vi "ReadEnricoData.vi"(0 "file path":path) -> (1 "Real Graph Enrico":cluster{"Signal":dbl[], "Signal":dbl[]}, 2 "Real Error bars":cluster{dbl[], dbl[]}(graph), 3 "Imaginary Graph Enrico":cluster{"Signal":dbl[], "Signal":dbl[]}, 4 "Imaginary Error bars":cluster{dbl[], dbl[]}(graph))   [LabVIEW 2011]
uses:
  <vilib>/Platform/storage/lvStorage.llb/_openStorageWithRootAutoDetect.vi
  <vilib>/Platform/storage/lvStorage.llb/xStorage/xStorageSupp/ErrorOut.vi
  <vilib>/Platform/storage/lvStorage.llb/_queryPropDateTime.vi
  <vilib>/Platform/storage/lvStorage.llb/_queryGenericObjects.vi
  <vilib>/Platform/storage/lvStorage.llb/_loadAllDouble.vi
  <vilib>/Platform/storage/Storage.llb/Get Object Info.vi
  <vilib>/Platform/storage/Storage.llb/__closeStorageFromObject.vi
  <vilib>/Platform/storage/lvStorage.llb/xStorage/Open Data Storage/Open Data Storage.xnode
  <vilib>/Platform/storage/lvStorage.llb/xStorage/Read Data/Read Data.xnode
  <vilib>/Platform/storage/lvStorage.llb/xStorage/Close Data Storage/Close Data Storage.xnode
panel:
  out "Imaginary Std":dbl[](array[numeric])
  out "Real std":dbl[](array[numeric])
  out "Imaginary":dbl[](array[numeric])
  out "Real":dbl[](array[numeric])
  out "WaveLength":dbl[](array[numeric])
  out "Signal":dbl[][](array[numeric])
  out "Double Charge Correction Flag":bool
  out "Concentration":dbl[][](array[numeric])
  out "Sizes":dbl[](array[numeric])
  out "error out":errorcluster
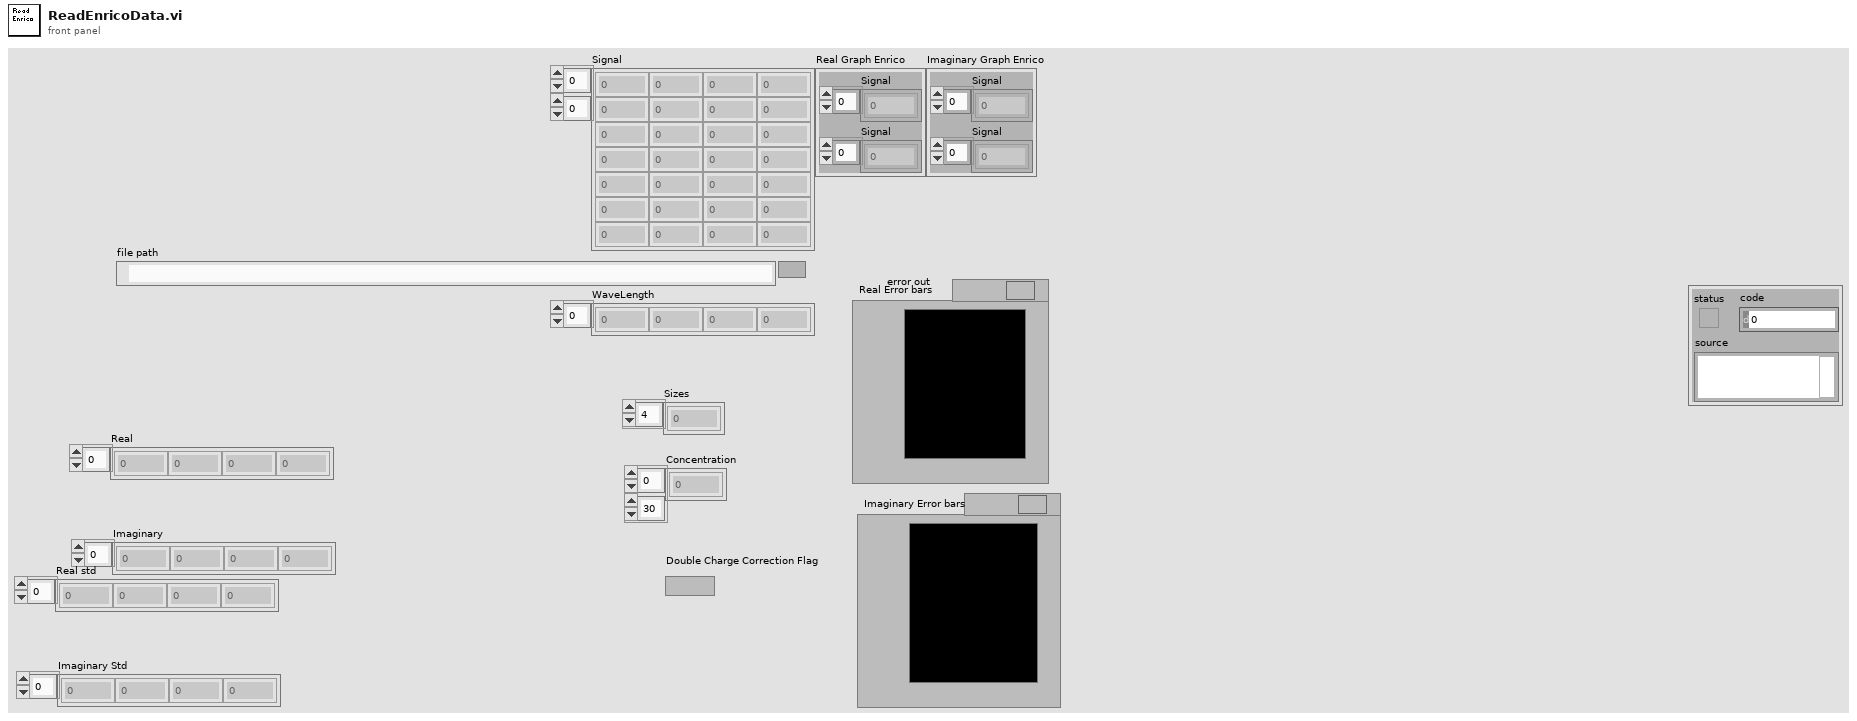
[diagram p1: front panel]
types:
  T1 = enum16{"open", "open or create", "create or replace", "create", "open (read only)"}
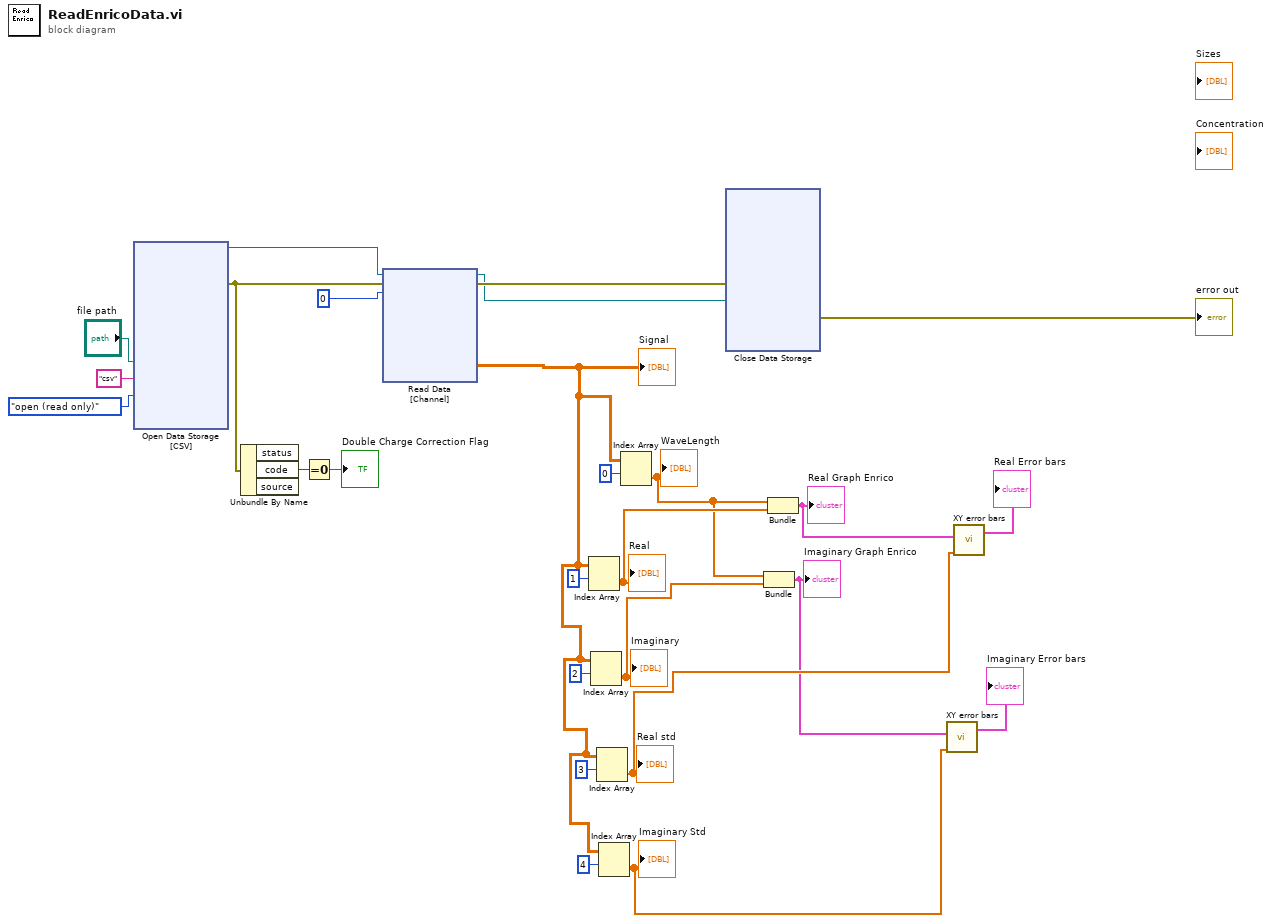
[diagram p0: block diagram]
diagram:
  n1 = xnode "Open Data Storage\n[CSV]"("file path"="file path", "DataPlugin name"="csv", "function (open:0)"=T1."open (read only)") -> ("storage refnum (file)"=w26:refnum<k20>, "error out"=w20:errorcluster)  [unwired: 2 in, 1 out]
  n2 = Unbundle By Name(w20) -> ("code"=w19:i32)  [unwired: 2 out]
  n3 = Equal To 0?(x=w19) -> (x = 0?=→"Double Charge Correction Flag":bool)
  n4 = xnode "Read Data\n[Channel]"("storage refnum (file)"=w26, "error in"=w20, "index"=0) -> ("Signal"=w10:dbl[][], "storage refnum (file) out"=w16:refnum<k20>, "error out"=w17:errorcluster)  [unwired: 1 in, 1 out]
  "Signal" <- w10
  n5 = Index Array(array=w10, index (row)=1) -> (element=w9:dbl[])  [unwired: 1 in]
  "Real" <- w9
  n6 = Index Array(array=w10, index (row)=2) -> (element=w8:dbl[])  [unwired: 1 in]
  "Imaginary" <- w8
  n7 = Index Array(array=w10, index (row)=3) -> (element=w5:dbl[])  [unwired: 1 in]
  "Real std" <- w5
  n8 = Index Array(array=w10, index (row)=4) -> (element=w2:dbl[])  [unwired: 1 in]
  "Imaginary Std" <- w2
  n9 = Index Array(array=w10, index (row)=0) -> (element=w7:dbl[])  [unwired: 1 in]
  "WaveLength" <- w7
  n10 = xnode "Close Data Storage\n"("error in (no error)"=w17, "storage refnum (file)"=w16) -> ("error out"=→"error out":errorcluster)  [unwired: 1 out]
  n11 = Bundle("Signal"=w7, "Signal"=w8) -> (w3:cluster{"Signal":dbl[], "Signal":dbl[]})  [unwired: 1 in]
  "Imaginary Graph Enrico" <- w3
  n12 = Bundle("Signal"=w7, "Signal"=w9) -> (w6:cluster{"Signal":dbl[], "Signal":dbl[]})  [unwired: 1 in]
  "Real Graph Enrico" <- w6
  n13 = call "XY error bars.vi"("XY plot"=w3, "Yerror"=w2) -> ("Y error bars"=→"Imaginary Error bars":cluster{dbl[], dbl[]})  [unwired: 6 in, 2 out]
  n14 = call "XY error bars.vi"("XY plot"=w6, "Yerror"=w5) -> ("Y error bars"=→"Real Error bars":cluster{dbl[], dbl[]})  [unwired: 6 in, 2 out]
